vi "DialogCreateClass.vi"(0 "ClassWriter in":refnum<class "ClassWriter.lvclass">, 1 "ProjectItem Refnum":refnum<vi>, 5 "error in (no error)":errorcluster) -> (14 "ClassWriter out":refnum<class "ClassWriter.lvclass">, 15 "Cancelled":bool, 16 "CreateClassData":T1, 17 "DesignPatternsToAddAfterCreation":string[](array[string]), 18 "ChangeProviderRequested":string, 19 "error out":errorcluster)   [LabVIEW 2020, in "ClassWriter.lvclass"]
uses:
  <resource>/Framework/Providers/Open_GDS/ClassProviders/Provider_BaseClassInterface/ClassWriter_class/ClassWriter.lvclass
  <resource>/Framework/Providers/Open_GDS/ClassProviders/Provider_BaseClassInterface/CreateClassData.ctl
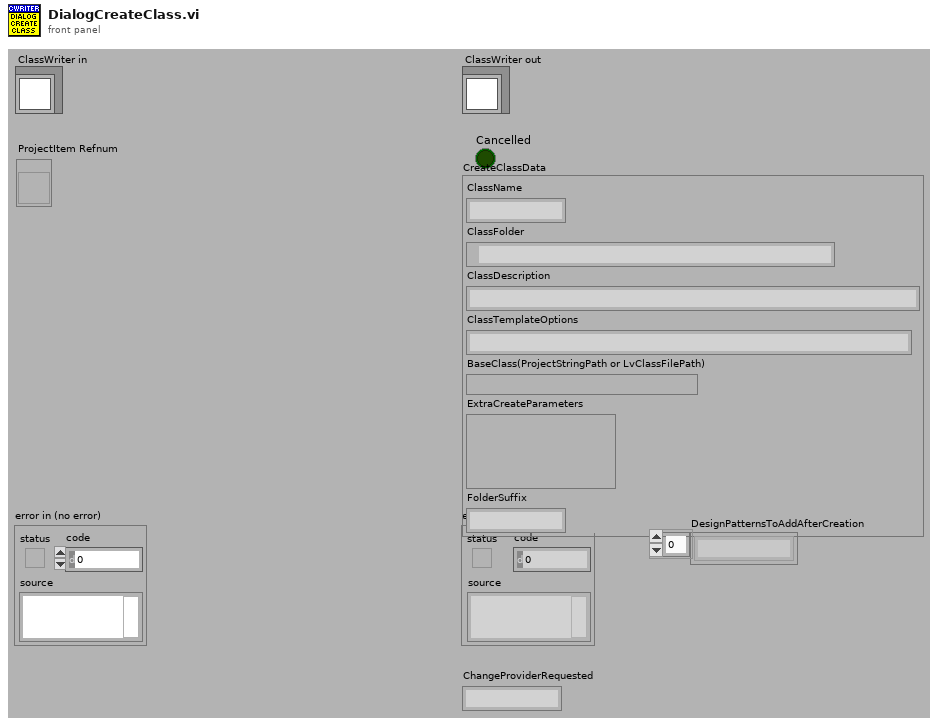
[diagram p1: front panel]
types:
  T1 = typedef "ClassWriter.lvclass/CreateClassData.ctl" = cluster{"ClassName":string, "ClassFolder":path, "ClassDescription":string, "ClassTemplateOptions":string, "BaseClass(ProjectStringPath or LvClassFilePath)":variant, "ExtraCreateParameters":variant, "FolderSuffix":string}
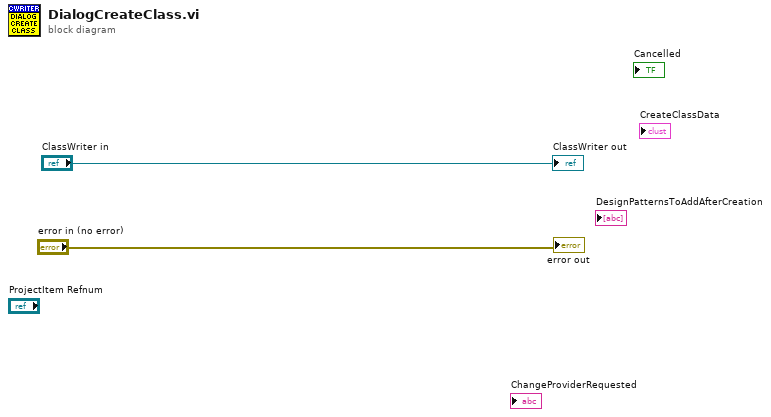
[diagram p0: block diagram]
diagram:
  "error out" <- "error in (no error)"
  "ClassWriter out" <- "ClassWriter in"
